vi "MAIN.vi"() -> ()   [LabVIEW 2024]
panel:
  out "Gate Exit":bool
  out "Gate Enter":bool
  in  "Timer 4":string
  in  "Timer 3":string
  in  "Timer 2":string
  in  "Timer 1":string
  out "4":bool
  out "3":bool
  out "2":bool
  out "1":bool
  # "Bay 1"
  # "Bay 2"
  # "Bay 3"
  # "Bay 4"
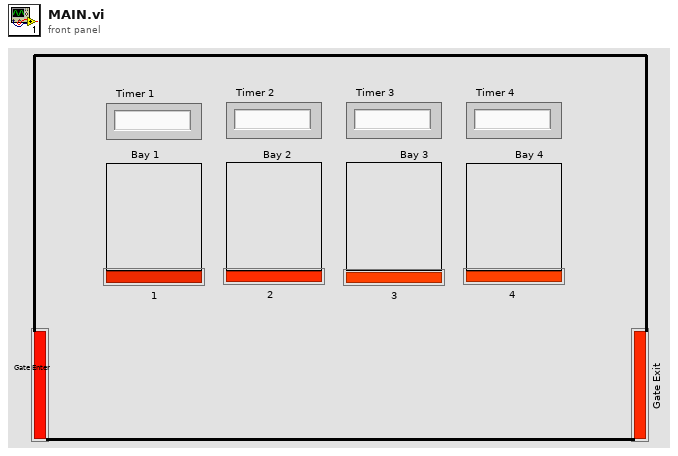
[diagram p1: front panel]
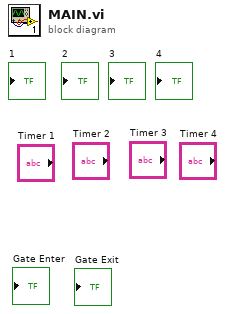
[diagram p0: block diagram]
diagram:
